vi "Get Epoch.vi"(10 "date time rec 2":T1) -> (0 "to epoch":T1, 2 "from epoch":T1)   [LabVIEW 2018]
uses:
  <vilib>/Utility/miscctls.llb/LVDateTimeRec.ctl
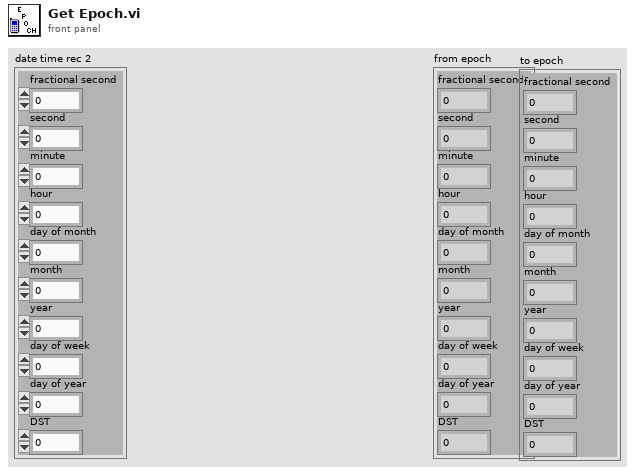
[diagram p1: front panel]
types:
  T1 = typedef "LVDateTimeRec.ctl" = cluster{"fractional second":dbl, "second":i32, "minute":i32, "hour":i32, "day of month":i32, "month":i32, "year":i32, "day of week":i32, "day of year":i32, "DST":i32}
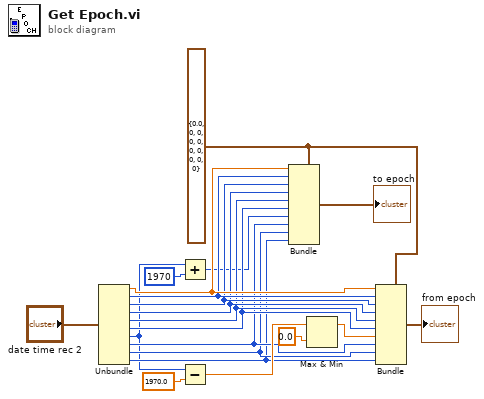
[diagram p0: block diagram]
diagram:
  w13 = T1 {"fractional second"=0.0, "second"=0, "minute"=0, "hour"=0, "day of month"=0, "month"=0, "year"=0, "day of week"=0, "day of year"=0, "DST"=0} ("date time rec 3")
  n1 = Unbundle("date time rec 2") -> ("fractional second"=w12:dbl, "second"=w11:i32, "minute"=w10:i32, "hour"=w9:i32, "day of month"=w8:i32, "month"=w7:i32, "year"=w2:i32, "day of week"=w6:i32, "day of year"=w5:i32, "DST"=w4:i32)
  n2 = Add(x=w2, y=1970) -> (x+y=w1:i32)
  n3 = Subtract(x=w2, y=1970.0) -> (x-y=w17:dbl)
  n4 = Bundle(cluster=w13, "fractional second"=w12, "second"=w11, "minute"=w10, "hour"=w9, "day of month"=w8, "month"=w7, "year"=w1, "day of week"=w6, "day of year"=w5, "DST"=w4) -> (→"to epoch":T1)
  n5 = Max & Min(x=w17, y=0.0) -> (max(x,y)=w16:dbl)  [unwired: 1 out]
  n6 = Bundle(cluster=w13, "fractional second"=w12, "second"=w11, "minute"=w10, "hour"=w9, "day of month"=w8, "month"=w7, "year"=w16, "day of week"=w6, "day of year"=w5, "DST"=w4) -> (→"from epoch":T1)
